vi "adler32.vi"(10 "ADLER-32 in (1)":u32=1 format="%08x", 11 "Data in":string) -> (3 "ADLER-32 out":u32 format="%08x")   [LabVIEW 2022 SP3, in "LabVIEW-Hashlib.lvlib"]
doc: "Calculates a 32-bit Cyclic Redundancy Check (CRC-32) for various algorithms."
uses:
  LabVIEW-Hashlib.lvlib
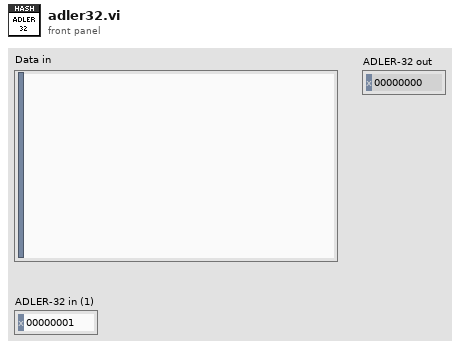
[diagram p1: front panel]
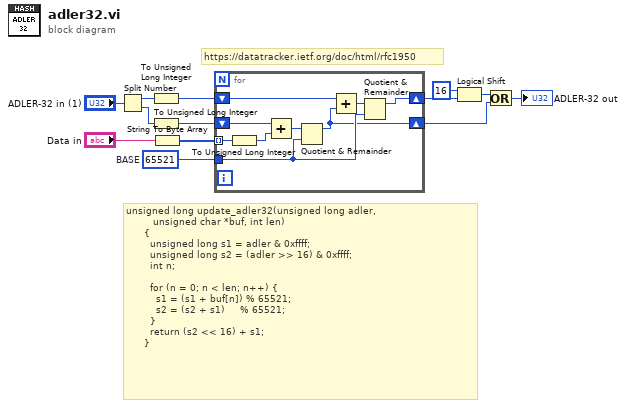
[diagram p0: block diagram]
diagram:
  w10 = u32 65521  # BASE
  # "unsigned long update_adler32(unsigned long adler,\n         unsigned char *buf, int len)\n      {\n        unsigned long s1 = adler & 0xffff;\n        unsigned long s2 = (adler >> 16) & 0xffff;\n        int n;\n\n        for (n = 0; n < len; n++) {\n          s1 = (s1 + buf[n]) % 65521;\n          s2 = (s2 + s1)     % 65521;\n        }\n        return (s2 << 16) + s1;\n      }"
  # "https://datatracker.ietf.org/doc/html/rfc1950"
  n1 = Split Number(x="ADLER-32 in (1)") -> (hi(x)=w12:u16, lo(x)=w11:u16)
  n2 = To Unsigned Long Integer(number=w12) -> (unsigned 32bit integer=w7:u32)
  n3 = To Unsigned Long Integer(number=w11) -> (unsigned 32bit integer=w6:u32)
  n4 = String To Byte Array(string="Data in") -> (unsigned byte array=w8:u8[])
  n5 = for {
    tunnel: w8 -> [w22] mode=indexing
    shift-right: [w15] -> w3
    shift-left: w6 -> [w21]
    shift-right: [w18] -> w5
    shift-left: w7 -> [w20]
    tunnel: w10 -> [w17]
    n6 = To Unsigned Long Integer(number=w22) -> (unsigned 32bit integer=w16:u32)
    n7 = Add(x=w21, y=w16) -> (x+y=w14:u32)
    n8 = Quotient & Remainder(x=w14, y=w17) -> (x-y*floor(x/y)=w15:u32)  [unwired: 1 out]
    n9 = Add(x=w20, y=w15) -> (x+y=w19:u32)
    n10 = Quotient & Remainder(x=w19, y=w17) -> (x-y*floor(x/y)=w18:u32)  [unwired: 1 out]
  }
  n11 = Logical Shift(y=i16 16, x=w5) -> (x << y=w2:u32)
  n12 = Or(x=w2, y=w3) -> (x .or. y?=→"ADLER-32 out":u32)
